vi "alertvisual.vi"() -> ()   [LabVIEW 2015]
uses:
  veloster/G_rio.vi
panel:
  out "Run":bool
  out "Auto":bool
  out "E - STOP":bool
  out "Camera":bool
  out "GPS":bool
  out "Laser":bool
  out "Steering":bool
  out "Gas/Brake":bool
  out "Control":bool
  out "CAN":bool
  out "Count GPS":i32
  out "Count CAN":i32
  out "Count Laser":i32
  out "Count camera":i32
  out "Count Control":i32
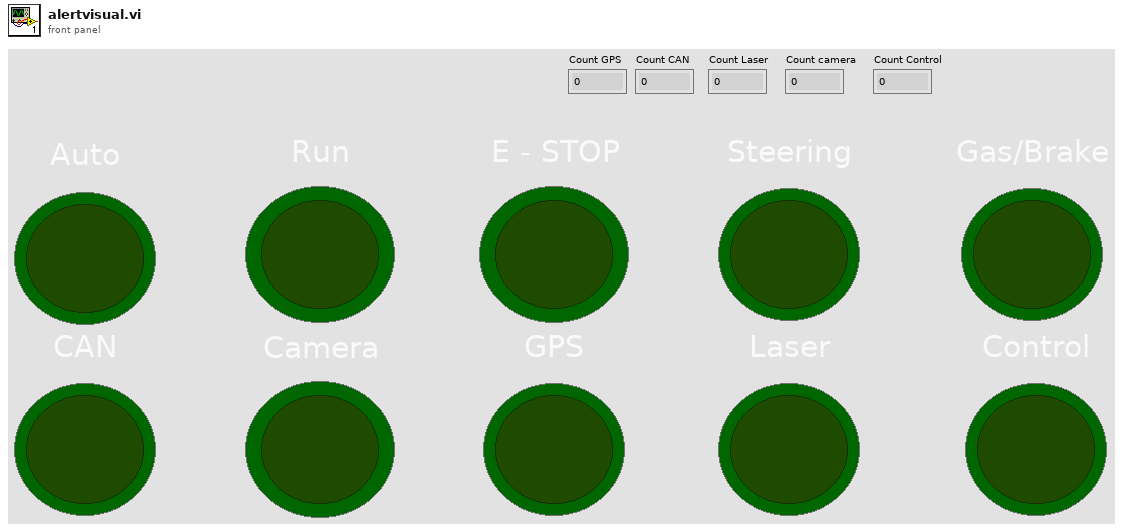
[diagram p1: front panel]
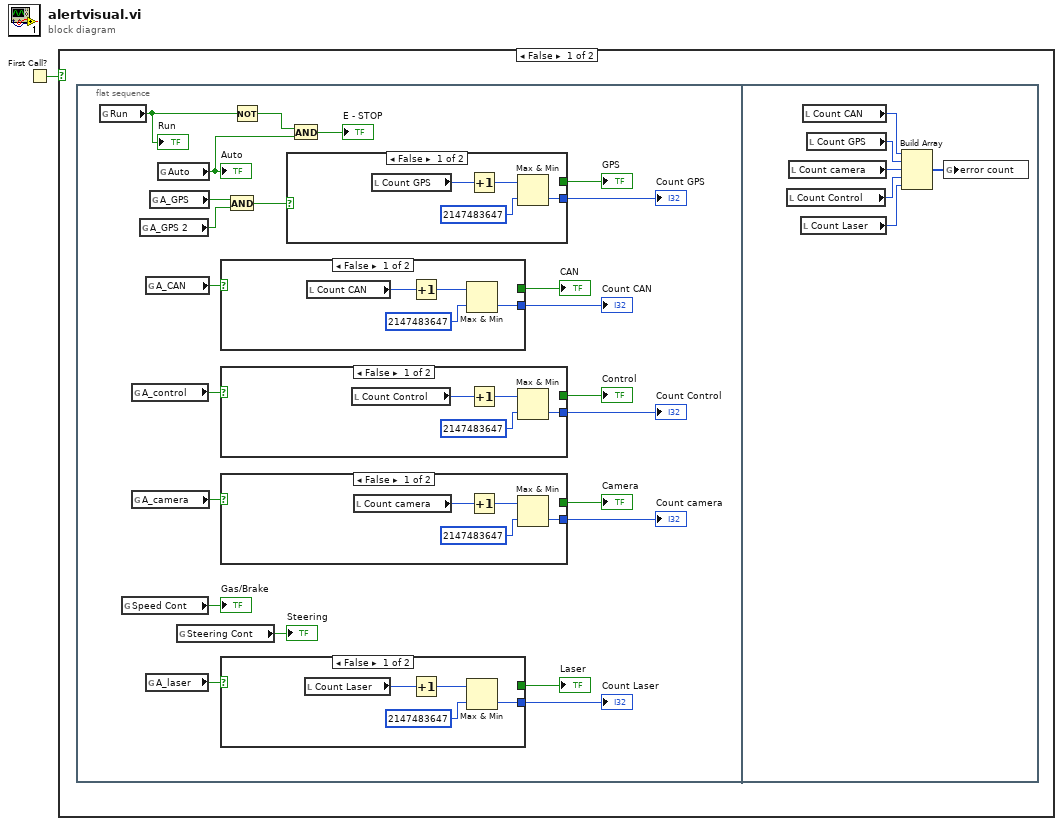
[diagram p0: block diagram]
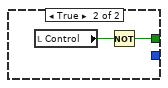
[diagram p2: hidden frame]
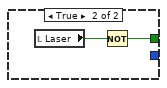
[diagram p3: hidden frame]
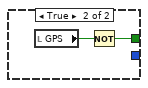
[diagram p4: hidden frame]
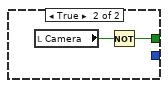
[diagram p5: hidden frame]
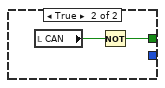
[diagram p6: hidden frame]
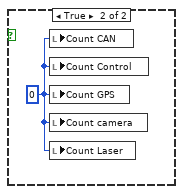
[diagram p7: hidden frame]
diagram:
  n1 = First Call?() -> (First Call?: T/F=w1:bool)
  n2 = case shown="False" w1 {
    frame False {
      n3 = flat-sequence {
        frame #0 {
          n4 = global read "G_rio.vi" "Run"() -> (w24:bool)
          "Run" <- w24
          n5 = global read "G_rio.vi" "Speed Cont"() -> (→"Gas/Brake":bool)
          n6 = global read "G_rio.vi" "A_control"() -> (w5:bool)
          n7 = global read "G_rio.vi" "A_camera"() -> (w18:bool)
          n8 = global read "G_rio.vi" "A_GPS 2"() -> (w3:bool)
          n9 = global read "G_rio.vi" "A_CAN"() -> (w20:bool)
          n10 = global read "G_rio.vi" "A_laser"() -> (w15:bool)
          n11 = global read "G_rio.vi" "A_GPS"() -> (w4:bool)
          n12 = global read "G_rio.vi" "Auto"() -> (w22:bool)
          "Auto" <- w22
          n13 = global read "G_rio.vi" "Steering Cont"() -> (→"Steering":bool)
          n14 = case shown="False" w20 {
            tunnel: [_ w53] -> w19
            tunnel: [w50 _] -> w10
            frame False {
              n15 = local read "Count CAN"() -> (w52:i32)
              n16 = Increment(x=w52) -> (x+1=w51:i32)
              n17 = Max & Min(x=w51, y=2147483647) -> (min(x,y)=w50:i32)  [unwired: 1 out]
            }
            frame True {
              n18 = local read "CAN"() -> (w54:bool)
              n19 = Not(x=w54) -> (.not. x?=w53:bool)
            }
          }
          "CAN" <- w19
          "Count CAN" <- w10
          n20 = case shown="False" w5 {
            tunnel: [_ w29] -> w6
            tunnel: [w25 _] -> w7
            frame False {
              n21 = local read "Count Control"() -> (w28:i32)
              n22 = Increment(x=w28) -> (x+1=w26:i32)
              n23 = Max & Min(x=w26, y=2147483647) -> (min(x,y)=w25:i32)  [unwired: 1 out]
            }
            frame True {
              n24 = local read "Control"() -> (w30:bool)
              n25 = Not(x=w30) -> (.not. x?=w29:bool)
            }
          }
          "Control" <- w6
          "Count Control" <- w7
          n26 = case shown="False" w18 {
            tunnel: [_ w47] -> w17
            tunnel: [w43 _] -> w11
            frame False {
              n27 = local read "Count camera"() -> (w46:i32)
              n28 = Increment(x=w46) -> (x+1=w44:i32)
              n29 = Max & Min(x=w44, y=2147483647) -> (min(x,y)=w43:i32)  [unwired: 1 out]
            }
            frame True {
              n30 = local read "Camera"() -> (w48:bool)
              n31 = Not(x=w48) -> (.not. x?=w47:bool)
            }
          }
          "Camera" <- w17
          "Count camera" <- w11
          n32 = case shown="False" w15 {
            tunnel: [_ w35] -> w14
            tunnel: [w31 _] -> w9
            frame False {
              n33 = local read "Count Laser"() -> (w34:i32)
              n34 = Increment(x=w34) -> (x+1=w33:i32)
              n35 = Max & Min(x=w33, y=2147483647) -> (min(x,y)=w31:i32)  [unwired: 1 out]
            }
            frame True {
              n36 = local read "Laser"() -> (w36:bool)
              n37 = Not(x=w36) -> (.not. x?=w35:bool)
            }
          }
          "Laser" <- w14
          "Count Laser" <- w9
          n38 = And(x=w4, y=w3) -> (x .and. y?=w2:bool)
          n39 = Not(x=w24) -> (.not. x?=w23:bool)
          n40 = case shown="False" w2 {
            tunnel: [_ w41] -> w16
            tunnel: [w37 _] -> w8
            frame False {
              n41 = local read "Count GPS"() -> (w40:i32)
              n42 = Increment(x=w40) -> (x+1=w39:i32)
              n43 = Max & Min(x=w39, y=2147483647) -> (min(x,y)=w37:i32)  [unwired: 1 out]
            }
            frame True {
              n44 = local read "GPS"() -> (w42:bool)
              n45 = Not(x=w42) -> (.not. x?=w41:bool)
            }
          }
          "GPS" <- w16
          "Count GPS" <- w8
          n46 = And(x=w23, y=w22) -> (x .and. y?=→"E - STOP":bool)
        }
        frame #1 {
          n47 = local read "Count Control"() -> (w57:i32)
          n48 = local read "Count camera"() -> (w58:i32)
          n49 = local read "Count Laser"() -> (w56:i32)
          n50 = local read "Count CAN"() -> (w60:i32)
          n51 = local read "Count GPS"() -> (w59:i32)
          n52 = Build Array(w60, w59, w58, w57, w56) -> (w55:i32[])
          n53 = global write "G_rio.vi" "error count"(w55) -> ()
        }
      }
    }
    frame True {
      w61 = 0 ("Count GPS")
      n54 = local write "Count CAN"(w61) -> ()
      n55 = local write "Count Control"(w61) -> ()
      n56 = local write "Count GPS"(w61) -> ()
      n57 = local write "Count camera"(w61) -> ()
      n58 = local write "Count Laser"(w61) -> ()
    }
  }
